vi "计算.vi"() -> ()   [LabVIEW 2016, in "斯坦道氨氮.lvlib"]
panel:
  in  "计算":bool
  out "计算结果":dbl caption="计算结果：" format="%#.6f"
  in  "吸光值":dbl caption="吸光值：" format="%#.6f"
  in  "曲线截距":dbl caption="曲线截距：" format="%#.6f"
  in  "曲线斜率":dbl caption="曲线斜率：" format="%#.6f"
  in  "二次多项式系数":dbl caption="二次多项式系数：" format="%#.6f"
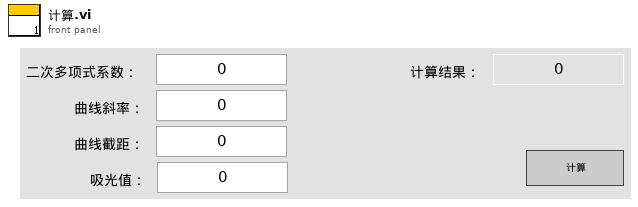
[diagram p1: front panel]
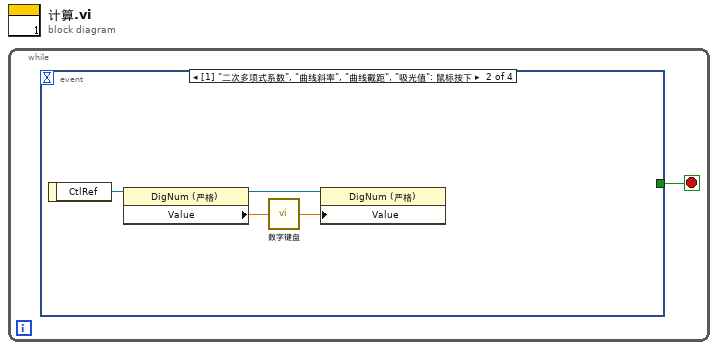
[diagram p0: block diagram]
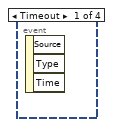
[diagram p2: hidden frame]
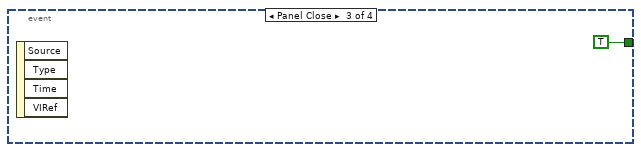
[diagram p3: hidden frame]
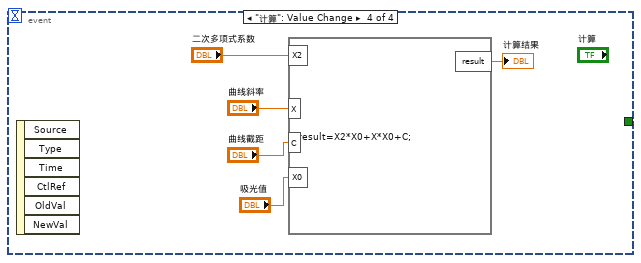
[diagram p4: hidden frame]
diagram:
  n1 = while {
    stop <- w1 stop-if-true
    n2 = event shown="[1] \"二次多项式系数\", \"曲线斜率\", \"曲线截距\", \"吸光值\": 鼠标按下" {
      selector: _ -> [_ _ _ _]
      dyn-events: _ -> [_ _ _ _]
      timeout: _ -> [_ _ _ _]
      tunnel: [_ _ TRUE _] -> w1
      event Timeout {
        n3 = event-data() -> ()  [unwired: 1 in, 3 out]
      }
      event "二次多项式系数", "曲线斜率", "曲线截距", "吸光值": Mouse Down {
        n4 = event-data() -> ("CtlRef"=w5:refnum<vi>)  [unwired: 1 in]
        n5 = property class="DigNum (严格)"(reference=w5) -> (reference out=w3:refnum<vi>, "Value"=w4:dbl)  [unwired: 1 in, 1 out]
        n6 = call "数字键盘.vi"("OldNumber"=w4) -> ("NewNumber"=w2:dbl)
        n7 = property class="DigNum (严格)"(reference=w3, "Value"=w2) -> ()  [unwired: 1 in, 2 out]
      }
      event Panel Close {
        n8 = event-data() -> ()  [unwired: 1 in, 4 out]
      }
      event "计算": Value Change {
        n9 = event-data() -> ()  [unwired: 1 in, 6 out]
        n10 = formula code="result=X2*X0+X*X0+C;"("X2"="二次多项式系数", "X"="曲线斜率", "C"="曲线截距", "X0"="吸光值") -> ("result"=→"计算结果":dbl)
      }
    }
  }
